vi "rx_ceEq.vi"(2 "preamble":cdb[](array[numeric])=[-0.7071067811865475+0.7071067811865476i, 0.7071067811865476+0.7071067811865475i, 0.7071067811865474-0.7071067811865477i, 0.7071067811865476+0.7071067811865475i, -0.7071067811865475+0.7071067811865476i, -0.7071067811865477-0.7071067811865475i, 0.7071067811865476+0.7071067811865475i, -0.7071067811865477-0.7071067811865475i, -0.7071067811865475+0.7071067811865476i, 0.7071067811865476+0.7071067811865475i, 0.7071067811865474-0.7071067811865477i, 0.7071067811865476+0.7071067811865475i, -0.7071067811865475+0.7071067811865476i, -0.7071067811865477-0.7071067811865475i, 0.7071067811865476+0.7071067811865475i, -0.7071067811865477-0.7071067811865475i, -0.7071067811865475+0.7071067811865476i, 0.7071067811865476+0.7071067811865475i, 0.7071067811865474-0.7071067811865477i, 0.7071067811865476+0.7071067811865475i, -0.7071067811865475+0.7071067811865476i, -0.7071067811865477-0.7071067811865475i, 0.7071067811865476+0.7071067811865475i, -0.7071067811865477-0.7071067811865475i, -0.7071067811865475+0.7071067811865476i, 0.7071067811865476+0.7071067811865475i, 0.7071067811865474-0.7071067811865477i, 0.7071067811865476+0.7071067811865475i, -0.7071067811865475+0.7071067811865476i, -0.7071067811865477-0.7071067811865475i, 0.7071067811865476+0.7071067811865475i, -0.7071067811865477-0.7071067811865475i, -0.7071067811865475+0.7071067811865476i, 0.7071067811865476+0.7071067811865475i, 0.7071067811865474-0.7071067811865477i, 0.7071067811865476+0.7071067811865475i, -0.7071067811865475+0.7071067811865476i, -0.7071067811865477-0.7071067811865475i, 0.7071067811865476+0.7071067811865475i, -0.7071067811865477-0.7071067811865475i, -0.7071067811865475+0.7071067811865476i, 0.7071067811865476+0.7071067811865475i, 0.7071067811865474-0.7071067811865477i, 0.7071067811865476+0.7071067811865475i, -0.7071067811865475+0.7071067811865476i, -0.7071067811865477-0.7071067811865475i, 0.7071067811865476+0.7071067811865475i, -0.7071067811865477-0.7071067811865475i, -0.7071067811865475+0.7071067811865476i, 0.7071067811865476+0.7071067811865475i, 0.7071067811865474-0.7071067811865477i, 0.7071067811865476+0.7071067811865475i, -0.7071067811865475+0.7071067811865476i, -0.7071067811865477-0.7071067811865475i, 0.7071067811865476+0.7071067811865475i, -0.7071067811865477-0.7071067811865475i, -0.7071067811865475+0.7071067811865476i, 0.7071067811865476+0.7071067811865475i, 0.7071067811865474-0.7071067811865477i, 0.7071067811865476+0.7071067811865475i, -0.7071067811865475+0.7071067811865476i, -0.7071067811865477-0.7071067811865475i, 0.7071067811865476+0.7071067811865475i, -0.7071067811865477-0.7071067811865475i], 3 "symbols":cdb[](array[numeric])) -> (0 "valid?":bool, 1 "eq symbols":cdb[](array[numeric]))   [LabVIEW 2014]
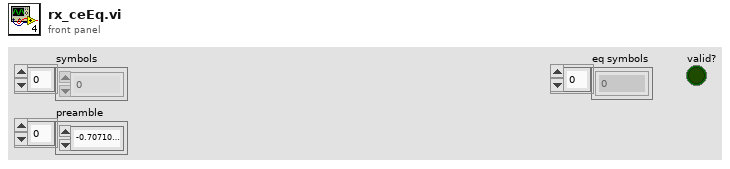
[diagram p1: front panel]
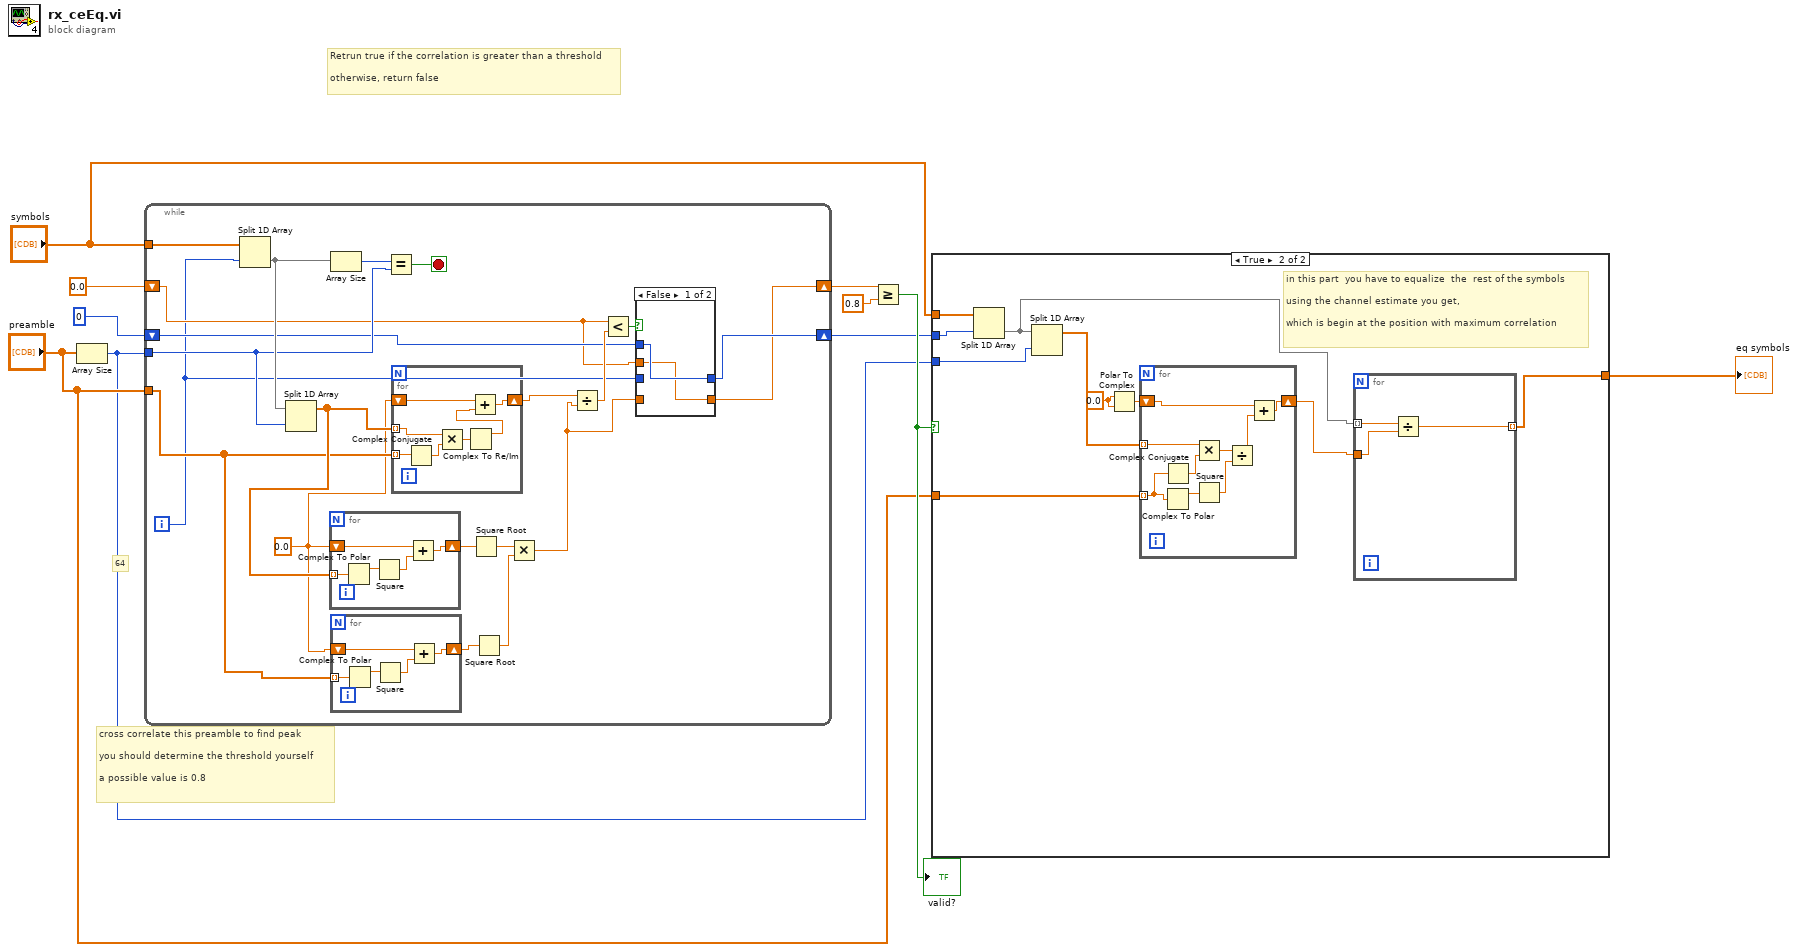
[diagram p0: block diagram]
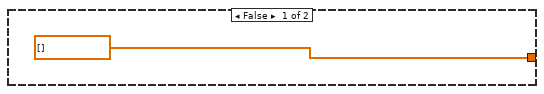
[diagram p3: hidden frame]
diagram:
  # "Retrun true if the correlation is greater than a threshold\n\notherwise, return false"
  # "cross correlate this preamble to find peak \n\nyou should determine the threshold yourself\n\na possible value is 0.8"
  # "64"
  n1 = Array Size(array="preamble") -> (size(s)=w1:i32)
  n2 = while {
    tunnel: "symbols" -> [w31]
    tunnel: w1 -> [w28]
    tunnel: "preamble" -> [w25]
    shift-right: [w13] -> w6
    shift-left: 0.0 -> [w17]
    shift-right: [w14] -> w2
    shift-left: 0 -> [w18]
    i -> [w16]
    stop <- w27 stop-if-true
    w12 = 0.0
    n3 = Split 1D Array(array=w31, index=w16) -> (second subarray=w29:cdb[])  [unwired: 1 out]
    n4 = Split 1D Array(array=w29, index=w28) -> (first subarray=w26:cdb[])  [unwired: 1 out]
    n5 = for {
      tunnel: w26 -> [w43] mode=indexing
      shift-right: [w44] -> w24
      shift-left: w12 -> [w45]
      n6 = Complex To Polar(r * e^(i*theta)=w43) -> (r=w42:dbl)  [unwired: 1 out]
      n7 = Square(x=w42) -> (x^2=w41:dbl)
      n8 = Add(x=w45, y=w41) -> (x+y=w44:dbl)
    }
    n9 = Array Size(array=w29) -> (size(s)=w30:i32)
    n10 = for {
      tunnel: w25 -> [w38] mode=indexing
      shift-right: [w39] -> w23
      shift-left: w12 -> [w40]
      n11 = Complex To Polar(r * e^(i*theta)=w38) -> (r=w37:dbl)  [unwired: 1 out]
      n12 = Square(x=w37) -> (x^2=w36:dbl)
      n13 = Add(x=w40, y=w36) -> (x+y=w39:dbl)
    }
    n14 = Equal?(x=w30, y=w28) -> (x = y?=w27:bool)
    n15 = for {
      tunnel: w26 -> [w50] mode=indexing
      tunnel: w25 -> [w52] mode=indexing
      shift-right: [w48] -> w11
      shift-left: w12 -> [w49]
      n16 = Complex Conjugate(1:w52) -> (0:w51:cdb)
      n17 = Multiply(x=w50, y=w51) -> (x*y=w47:cdb)
      n18 = Complex To Re/Im(x + iy=w47) -> (x=w46:dbl)  [unwired: 1 out]
      n19 = Add(x=w49, y=w46) -> (x+y=w48:dbl)
    }
    n20 = Square Root(x=w24) -> (sqrt(x)=w22:dbl)
    n21 = Square Root(x=w23) -> (sqrt(x)=w21:dbl)
    n22 = Multiply(x=w22, y=w21) -> (x*y=w15:dbl)
    n23 = Divide(x=w11, y=w15) -> (x/y=w19:dbl)
    n24 = Less?(x=w17, y=w19) -> (x < y?=w20:bool)
    n25 = case shown="False" w20 {
      tunnel: w18 -> [w33 _]
      tunnel: w17 -> [w32 _]
      tunnel: w16 -> [_ w35]
      tunnel: w15 -> [_ w34]
      tunnel: [w33 w35] -> w14
      tunnel: [w32 w34] -> w13
      frame False {
      }
      frame True {
      }
    }
  }
  n26 = Greater Or Equal?(x=w6, y=0.8) -> (x >= y?=w5:bool)
  "valid?" <- w5
  n27 = case shown="True" w5 {
    tunnel: [cdb[] [] w54] -> w10
    tunnel: "symbols" -> [_ w63]
    tunnel: "preamble" -> [_ w59]
    tunnel: w2 -> [_ w62]
    tunnel: w1 -> [_ w61]
    frame False {
    }
    frame True {
      w58 = 0.0
      # "in this part  you have to equalize  the  rest of the symbols\n\nusing the channel estimate you get, \n\nwhich is begin at the position with maximum correlation"
      n28 = Split 1D Array(array=w63, index=w62) -> (second subarray=w56:cdb[])  [unwired: 1 out]
      n29 = Split 1D Array(array=w56, index=w61) -> (first subarray=w60:cdb[])  [unwired: 1 out]
      n30 = Polar To Complex(1:w58, 2:w58) -> (0:w57:cdb)
      n31 = for {
        tunnel: w60 -> [w74] mode=indexing
        tunnel: w59 -> [w73] mode=indexing
        shift-right: [w67] -> w55
        shift-left: w57 -> [w69]
        n32 = Complex Conjugate(1:w73) -> (0:w75:cdb)
        n33 = Complex To Polar(r * e^(i*theta)=w73) -> (r=w72:dbl)  [unwired: 1 out]
        n34 = Multiply(x=w74, y=w75) -> (x*y=w71:cdb)
        n35 = Square(x=w72) -> (x^2=w70:dbl)
        n36 = Divide(x=w71, y=w70) -> (x/y=w68:cdb)
        n37 = Add(x=w69, y=w68) -> (x+y=w67:cdb)
      }
      n38 = for {
        tunnel: w56 -> [w66] mode=indexing
        tunnel: w55 -> [w65]
        tunnel: [w64] -> w54 mode=indexing
        n39 = Divide(x=w66, y=w65) -> (x/y=w64:cdb)
      }
    }
  }
  "eq symbols" <- w10
